vi "Actor Core.vi.BACKUP.11232.vi"(8 "error in":errorcluster, 11 "Data Logger in":refnum<class "Data Logger.lvclass">) -> (0 "error out":errorcluster, 3 "Actor out":refnum<class "Actor.lvclass">)   [LabVIEW 2013, in "Data Logger.lvlib" / "Data Logger.lvclass"]
doc: "(<B>Filename</B>: Actor Framework.lvlib:Actor.lvclass:Actor Core.vi)\n\nReceives messages to the actor, reacts to them, and initiates any error handling that may shut the actor down.\n\nDescendant classes may override this VI to append parallel tasks for the actor to complete while it handles messages. Overrides use the Call Parent Method node."
uses:
  Data Logger.lvclass
  <vilib>/ActorFramework/Actor/Actor.lvclass
  <vilib>/express/express signal manip/GetorSetDDTAttributes/Set DDT Attributes/Set DDT Properties.xnode
  Display Panel/Abstract Display Messages/Write State Ref Msg/Write State Ref Msg.lvclass
  Display Panel/Abstract Display/Control 1.ctl
  <vilib>/express/express shared/transition.llb/Dynamic To Waveform Array.vi
  <vilib>/express/express signal manip/GetorSetDDTAttributes/Set DDT Attributes/SetT0.vi
  <vilib>/express/express shared/transition.llb/Waveform Array To Dynamic.vi
panel:
  out "Number of sent":i32
  in  "States":T1
  out "floor(x/y)":dbl
  out "Elapsed Time (s)":dbl format="%<%H:%M:%S>t"
  out "nearest integer value":dbl
  out "x = 0?":bool
  out "x-y*floor(x/y)":dbl
  in  "Parent i":i32
  out "Waveform Chart":dbl(graph)
  out "Scalar":dbl
  in  "Waveform Graph 2":dynamicdata(graph)
  out "i":i32
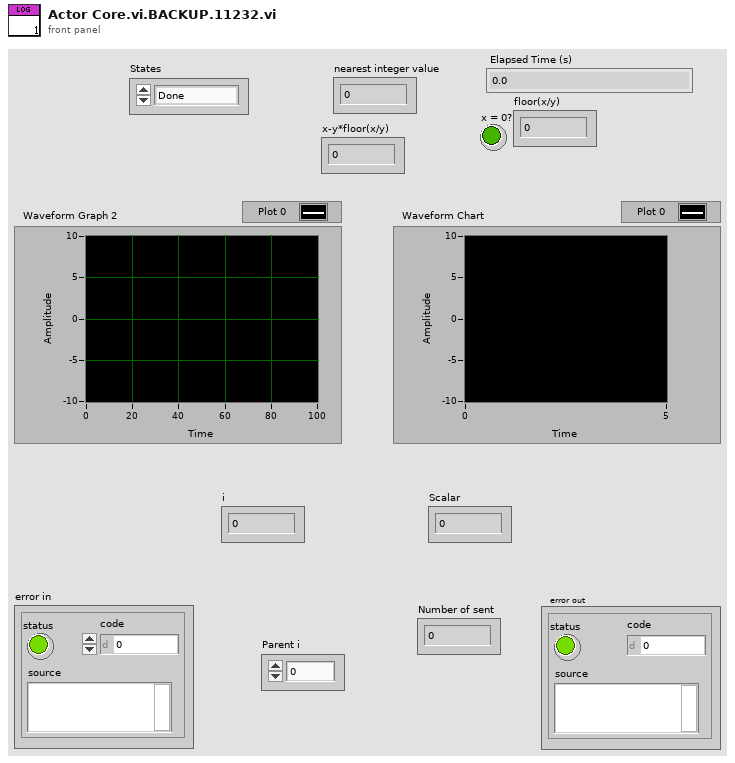
[diagram p1: front panel]
types:
  T1 = typedef "Display Panel.lvlib/Abstract Display.lvclass/Control 1.ctl" = enum16{"Done", "Warming", "Measuring"}
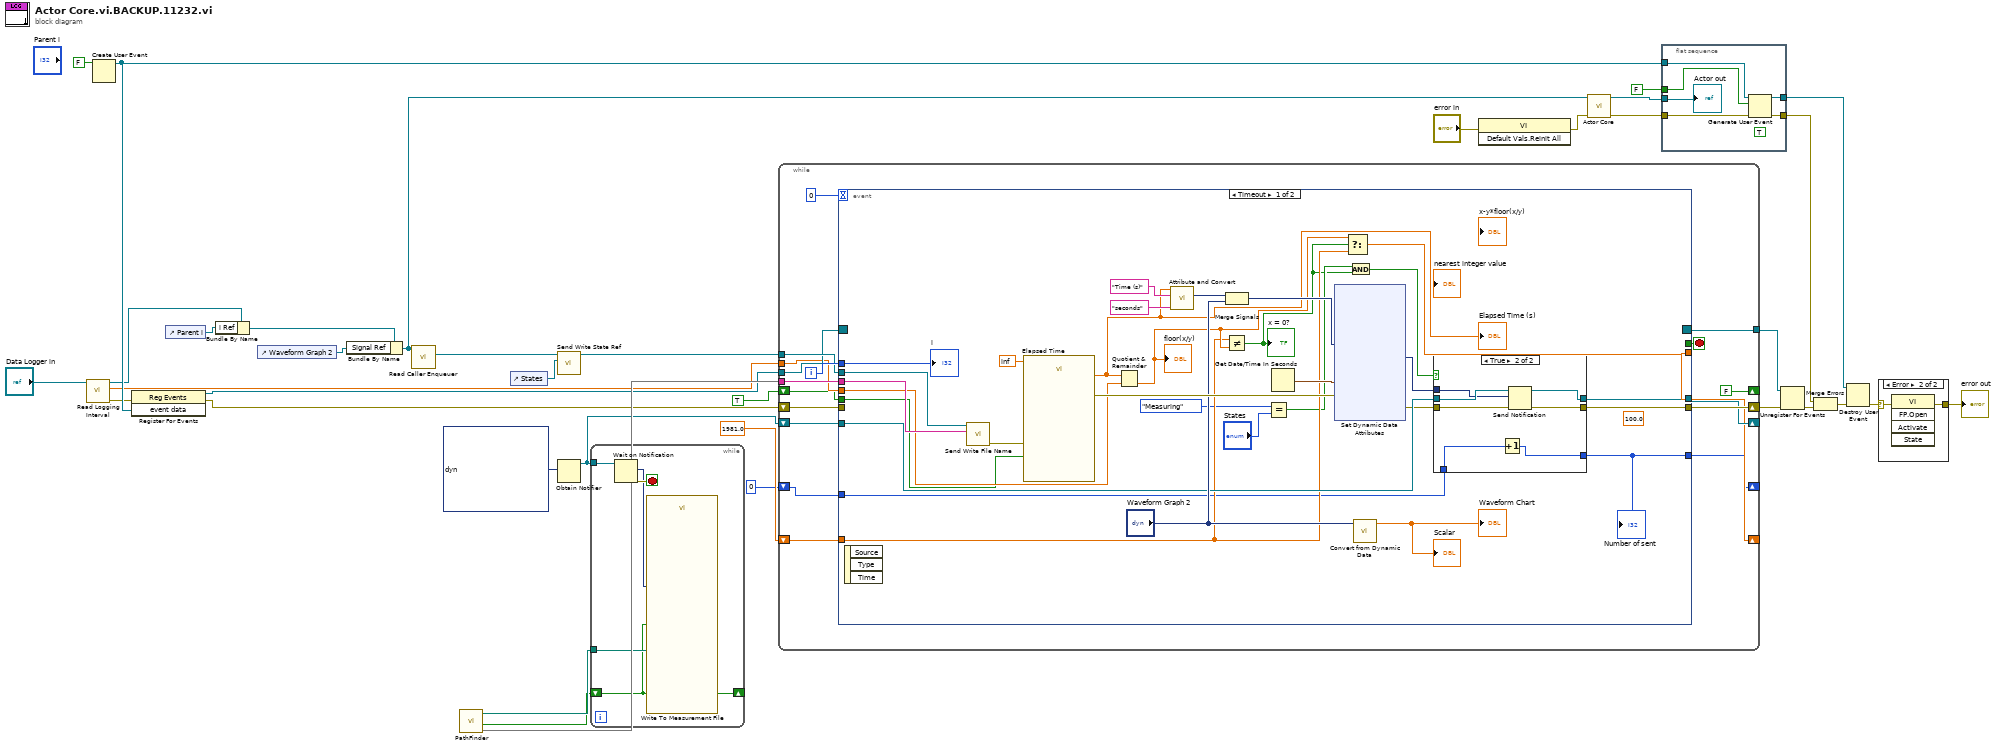
[diagram p0: block diagram]
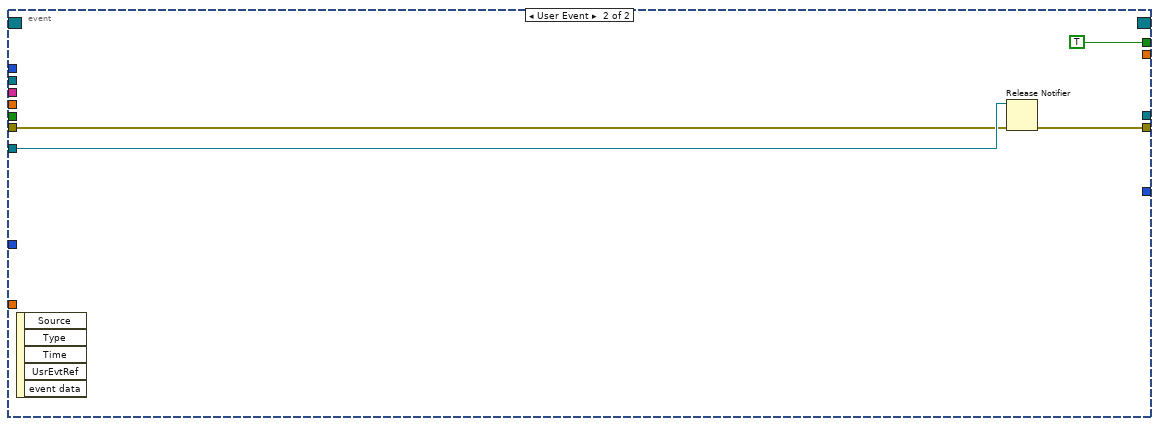
[diagram p4: hidden frame]
diagram:
  n1 = call "Read Logging Interval.vi"("Data Logger in"="Data Logger in") -> ("error out"=w7:errorcluster, "Logging Interval"=w8:dbl, "Data Logger out"=w9:refnum<class "Data Logger.lvclass">)  [unwired: 8 in]
  n2 = Create User Event(user event datatype=FALSE ("event data")) -> (user event=w19:refnum<user-event>)  [unwired: 1 in, 1 out]
  n3 = register-events(error in=w7, w19) -> (reference out=w18:refnum<event-registration>, error out=w15:errorcluster)  [unwired: 1 in]
  n4 = control-ref of="Parent i"() -> (w30:refnum<vi>)
  n5 = Bundle By Name(cluster=w9, "i Ref"=w30) -> (w31:refnum<class "Data Logger.lvclass">)
  n6 = control-ref of="Waveform Graph 2"() -> (w35:refnum<vi>)
  n7 = Bundle By Name(cluster=w31, "Signal Ref"=w35) -> (w27:refnum<class "Data Logger.lvclass">)
  n8 = call <vilib>:"Read Caller Enqueuer.vi"("Actor"=w27) -> ("Caller Enqueuer"=w3:refnum<class "Message Enqueuer.lvclass">)  [unwired: 10 in]
  n9 = call "PathFinder.vi"() -> (0:w26, "Save?"=w22:bool, "selected path"=w23:path)  [unwired: 9 in]
  n10 = control-ref of="States"() -> (w4:refnum<vi>)
  n11 = call "Send Write State Ref.vi"("State Ref"=w4, "Message Enqueuer"=w3) -> ("Message Enqueuer out"=w2:refnum<class "Message Enqueuer.lvclass">)  [unwired: 8 in, 1 out]
  n12 = Obtain Notifier(notification data type=dynamicdata [] ("Waveform Graph 3")) -> (notifier out=w25:refnum<notifier>)  [unwired: 3 in, 2 out]
  n13 = while {
    tunnel: w25 -> [w41]
    tunnel: w23 -> [w38]
    shift-right: [w37] -> _
    shift-left: w22 -> [w37]
    stop <- w40 stop-if-true
    n14 = Wait on Notification(notifier=w41) -> (notification=w39:dynamicdata, error out=w40:errorcluster)  [unwired: 1 in, 4 out]
    n15 = call "Write To Measurement File"("Signals"=w39, "Enable"=w37, "Filename"=w38) -> ()  [unwired: 14 in, 3 out]
  }
  n16 = while {
    tunnel: w2 -> [w58]
    tunnel: w26 -> [w57]
    tunnel: w18 -> [w54]
    tunnel: [w53] -> w17
    shift-right: [w50] -> _
    shift-left: w25 -> [w56]
    shift-right: [w55] -> w14
    shift-left: w15 -> [w49]
    tunnel: w8 -> [w48]
    shift-right: [FALSE] -> _
    shift-left: TRUE -> [w47]
    shift-right: [w44] -> _
    shift-left: 1981.0 -> [w45]
    shift-right: [w42] -> _
    shift-left: 0 -> [w43]
    i -> [w59]
    stop <- w51 stop-if-true
    n17 = event shown="[0] Timeout" {
      selector: w54 -> [_ _]
      dyn-events: [_ _] -> w53
      timeout: 0 -> [_ _]
      tunnel: w59 -> [w90 _]
      tunnel: w58 -> [w89 _]
      tunnel: w57 -> [w88 _]
      tunnel: w56 -> [w77 w117]
      tunnel: [w75 w115] -> w55
      tunnel: [_ TRUE] -> w51
      tunnel: [w74 _] -> w50
      tunnel: w49 -> [_ w116]
      tunnel: w48 -> [w72 _]
      tunnel: w47 -> [w71 _]
      tunnel: w45 -> [w67 _]
      tunnel: [w69 _] -> w44
      tunnel: w43 -> [w61 _]
      tunnel: [w60 _] -> w42
      event Timeout {
        (unwired) 100.0 ("y")
        n18 = event-data() -> ()  [unwired: 1 in, 3 out]
        n19 = call "Send Write File Name.vi"("File Name"=w88, "Message Enqueuer"=w89) -> ("error out"=w78:errorcluster)  [unwired: 8 in, 1 out]
        n20 = call "Elapsed Time"("Time Target (s)"=inf, "Reset"=w71, "error in (no error)"=w78) -> ("Elapsed Time (s)"=w70:dbl, "error out"=w80:errorcluster)  [unwired: 9 in, 6 out]
        "Elapsed Time (s)" <- w70
        n21 = Quotient & Remainder(x=w70, y=w72) -> (floor(x/y)=w68:dbl)  [unwired: 1 out]
        "floor(x/y)" <- w68
        n22 = call "Attribute and Convert.vi"("Unit"="seconds", "Signal Name"="Time (s)", "Number in"=w70) -> ("Dynamic Signal Out"=w85:dynamicdata)  [unwired: 8 in]
        n23 = Merge Signals(w85, "Waveform Graph 2") -> (w83:dynamicdata)
        n24 = Not Equal?(x=w67, y=w68) -> (x != y?=w63:bool)
        "x = 0?" <- w63
        n25 = Equal?(x=Control_1."Measuring" ("States 2"), y="States") -> (x = y?=w64:bool)
        n26 = Get Date/Time In Seconds() -> (seconds since 1Jan1904=w87:timestamp)
        n27 = xnode "Set Dynamic Data Attributes"("Signals In"=w83, "Timestamp"=w87, "error in"=w80) -> ("Signals Out"=w76:dynamicdata, "error out"=w73:errorcluster)  [unwired: 1 in]
        n28 = Select(t=w68, s=w63, f=w67) -> (s? t:f=w69:dbl)
        n29 = And(x=w64, y=w63) -> (x .and. y?=w62:bool)
        n30 = call "Convert from Dynamic Data"("Dynamic Data Type"="Waveform Graph 2") -> ("Scalar"=→"Scalar" →"Waveform Chart":dbl)  [unwired: 3 in]
        n31 = case shown="True" w62 {
          tunnel: w77 -> [w93 w100]
          tunnel: w76 -> [_ w99]
          tunnel: [w92 w98] -> w75
          tunnel: [w93 w97] -> w74
          tunnel: w73 -> [w92 w96]
          tunnel: w61 -> [w91 w95]
          tunnel: [w91 w94] -> w60
          frame False {
          }
          frame True {
            n32 = Increment(x=w95) -> (x+1=w94:i32)
            n33 = Send Notification(notification=w99, notifier=w100, error in (no error)=w96) -> (notifier out=w97:refnum<notifier>, error out=w98:errorcluster)
          }
        }
        "Number of sent" <- w60
        "i" <- w90
      }
      event User Event {
        n34 = event-data() -> ()  [unwired: 1 in, 5 out]
        n35 = Release Notifier(notifier=w117, error in (no error)=w116) -> (error out=w115:errorcluster)  [unwired: 3 out]
      }
    }
  }
  n36 = invoke class="VI" method="Default Vals.Reinit All"(error in="error in") -> (error out=w28:errorcluster)  [unwired: 2 in, 2 out]
  n37 = call-parent "Actor Core.vi"("error in"=w28, "Actor in"=w27) -> ("error out"=w32:errorcluster, "Actor out"=w36:refnum<class "Actor.lvclass">)  [unwired: 8 in]
  n38 = flat-sequence {
    tunnel: w36 -> [w124]
    tunnel: FALSE ("event data") -> [w119]
    tunnel: w32 -> [w121]
    tunnel: [w123] -> w21
    tunnel: [w122] -> w11
    tunnel: w19 -> [w120]
    frame #0 {
      (unwired) TRUE ("Stop Button")
      n39 = Generate User Event(user event=w120, event data cluster=w119, error in=w121) -> (user event out=w123:refnum<user-event>, error out=w122:errorcluster)  [unwired: 1 in]
      "Actor out" <- w124
    }
  }
  n40 = Unregister For Events(event registration refnum=w17, error in=w14) -> (error out=w12:errorcluster)
  n41 = Merge Errors(w11, w12) -> (w13:errorcluster)
  n42 = Destroy User Event(user event=w21, error in=w13) -> (error out=w16:errorcluster)
  n43 = case shown="Error" w16 {
    selector: w16 -> [w125 w127]
    tunnel: [w125 w126] -> w33
    frame No Error {
    }
    frame Error {
      n44 = invoke class="VI" method="FP.Open"(error in=w127) -> (error out=w126:errorcluster)  [unwired: 4 in, 4 out]
    }
  }
  "error out" <- w33
